vi "localArquivo.vi"(7 "quantidadeDeArquivos":i16, 8 "nAtualDoArquivo":i16, 9 "extensão":string, 10 "Nome do arquivo":string, 11 "Local":path) -> (3 "Path":path)   [LabVIEW 2012]
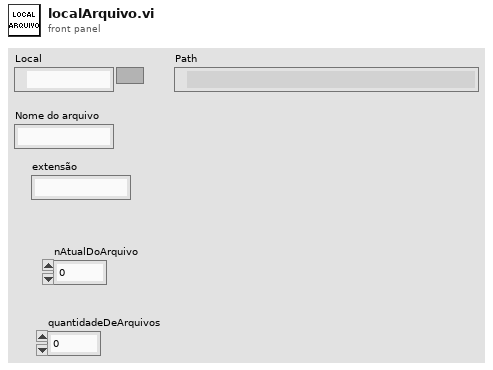
[diagram p1: front panel]
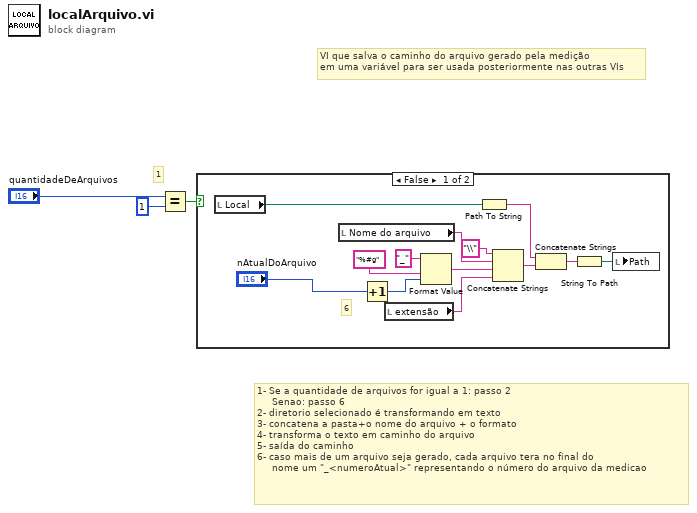
[diagram p0: block diagram]
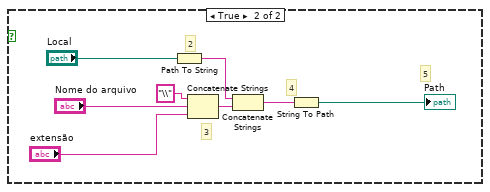
[diagram p2: hidden frame]
diagram:
  # "VI que salva o caminho do arquivo gerado pela medição\nem uma variável para ser usada posteriormente nas outras VIs"
  # "1- Se a quantidade de arquivos for igual a 1: passo 2\n     Senao: passo 6\n2- diretorio selecionado é transformando em texto \n3- concatena a pasta+o nome do arquivo + o formato\n4- transforma o texto em caminho do arquivo\n5- saída do caminho\n6- caso mais de um arquivo seja gerado, cada arquivo tera no final do\n     nome um \"_<numeroAtual>\" representando o número do arquivo da medicao"
  # "1"
  n1 = Equal?(x="quantidadeDeArquivos", y=i64 1) -> (x = y?=w2:bool)
  n2 = case shown="False" w2 {
    frame False {
      # "6"
      n3 = local read "Local"() -> (w13:path)
      n4 = local read "Nome do arquivo"() -> (w12:string)
      n5 = Increment(x="nAtualDoArquivo") -> (x+1=w8:i16)
      n6 = local read "extensão"() -> (w10:string)
      n7 = Format Value(string ("")="_", format string="%#g", value (0)=w8) -> (output string=w7:string)
      n8 = Path To String(path=w13) -> (string=w15:string)
      n9 = Concatenate Strings("\\" ("string"), w12, w7, w10) -> (w16:string)
      n10 = Concatenate Strings(w15, w16) -> (w14:string)
      n11 = String To Path(string=w14) -> (path=w6:path)
      n12 = local write "Path"(w6) -> ()
    }
    frame True {
      # "5"
      # "4"
      # "3"
      # "2"
      n13 = Path To String(path="Local") -> (string=w22:string)
      n14 = Concatenate Strings("\\", "Nome do arquivo", "extensão") -> (w23:string)
      n15 = Concatenate Strings(w22, w23) -> (w21:string)
      n16 = String To Path(string=w21) -> (path=→"Path":path)
    }
  }
